vi "GT Get Home Prm.vi"(8 "error in (no error)":errorcluster caption="错误输入（无错误）", 9 "pHomePrm":T1, 10 "axis":i16, 11 "cardNum":i16) -> (0 "error out":errorcluster caption="错误输出", 1 "pHomePrm out":T1, 3 "function return":i16)   [LabVIEW 2014, in "gts.lvlib"]
doc: "GT_API GT_GetHomePrm(short cardNum,short axis,THomePrm *pHomePrm);"
uses:
  gts.lvlib
  gts.dll
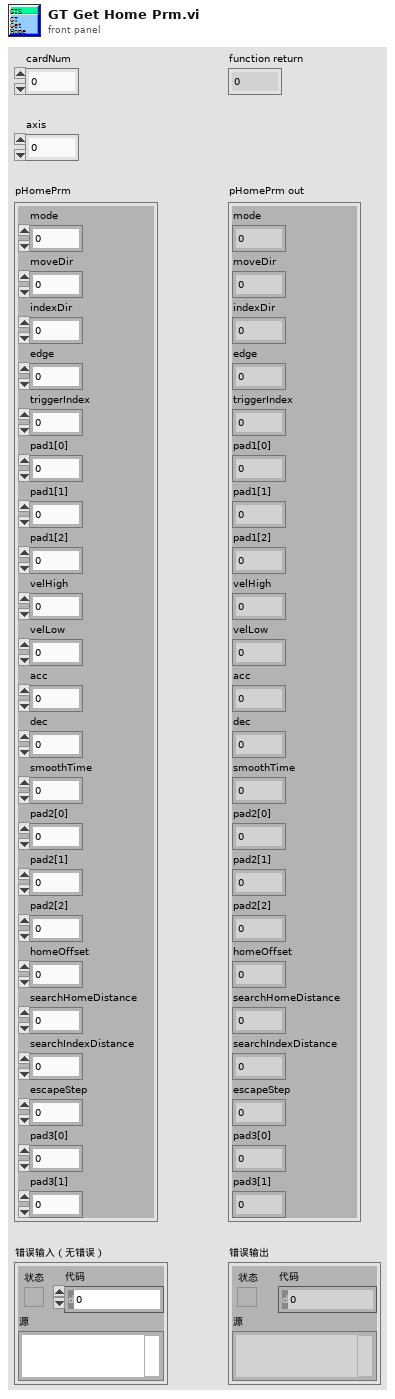
[diagram p1: front panel]
types:
  T1 = cluster{"mode":i16, "moveDir":i16, "indexDir":i16, "edge":i16, "triggerIndex":i16, "pad1[0]":i16, "pad1[1]":i16, "pad1[2]":i16, "velHigh":dbl, "velLow":dbl, "acc":dbl, "dec":dbl, "smoothTime":i16, "pad2[0]":i16, "pad2[1]":i16, "pad2[2]":i16, "homeOffset":i32, "searchHomeDistance":i32, "searchIndexDistance":i32, "escapeStep":i32, "pad3[0]":i32, "pad3[1]":i32}
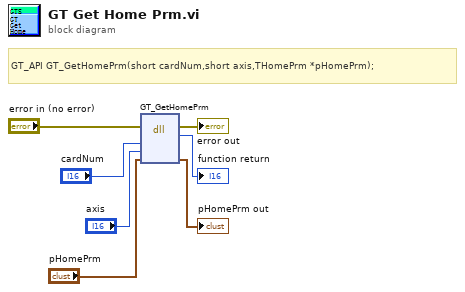
[diagram p0: block diagram]
diagram:
  # "GT_API GT_GetHomePrm(short cardNum,short axis,THomePrm *pHomePrm);"
  n1 = dll-call lib="PTH2>abs F.多卡库-控制卡基本运动例程(labview)gts.*" fn="GT_GetHomePrm"(error in="error in (no error)", "cardNum"="cardNum", "axis"="axis", "pHomePrm"="pHomePrm") -> (error out=→"error out":errorcluster, →"function return":i16, "pHomePrm"=→"pHomePrm out":T1)  [unwired: 4 in, 1 out]
